vi "Save to File 2D.vi"(8 "error in":errorcluster, 9 "New file?":bool, 10 "2D data":string[][](array[string]), 11 "CSV in":refnum<class "CSV.lvclass">) -> (0 "error out":errorcluster, 3 "CSV out":refnum<class "CSV.lvclass">)   [LabVIEW 2017, in "Reports.lvlib" / "CSV.lvclass"]
doc: "This method write 2D str Array\nto file with predefined Filepath"
uses:
  CSV.lvclass
  CSV.lvclass/CSV.ctl
  <vilib>/Utility/file.llb/Write Delimited Spreadsheet (string).vi
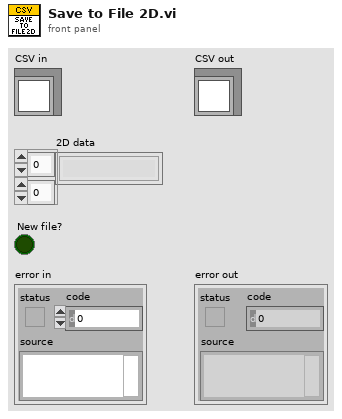
[diagram p1: front panel]
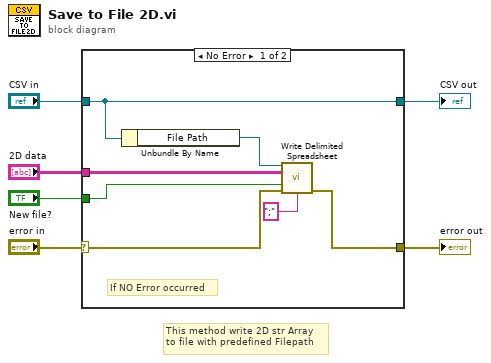
[diagram p0: block diagram]
diagram:
  # "This method write 2D str Array\nto file with predefined Filepath"
  n1 = case shown="No Error" "error in" {
    selector: "error in" -> [w10 w15]
    tunnel: [w9 w15] -> w5
    tunnel: [w8 w14] -> w3
    tunnel: "CSV in" -> [w8 w14]
    tunnel: "2D data" -> [w12 _]
    tunnel: "New file?" -> [w11 _]
    frame No Error {
      # "If NO Error occurred"
      n2 = Unbundle By Name(w8) -> ("File Path"=w7:path)
      n3 = call-poly <vilib>:"Write Delimited Spreadsheet.vi"("file path (dialog if empty)"=w7, "2D data"=w12, "append to file? (new file:F)"=w11, "error in (no error)"=w10, "delimiter (\\t)"=";" ("delimiter (\\t)")) -> ("error out"=w9:errorcluster)  [unwired: 9 in, 1 out]
    }
    frame Error {
    }
  }
  "error out" <- w5
  "CSV out" <- w3
